vi "数值至码管数组转换.vi"(9 "小数位数":u8, 10 "显示位数":u8=6, 11 "数值":dbl format="%06.3f") -> (3 "数组":u16[](array[numeric]))   [LabVIEW 2013, in "数码管.xctl"]
panel:
  out "子字符串":string
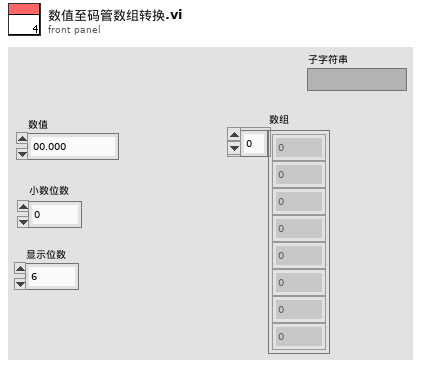
[diagram p1: front panel]
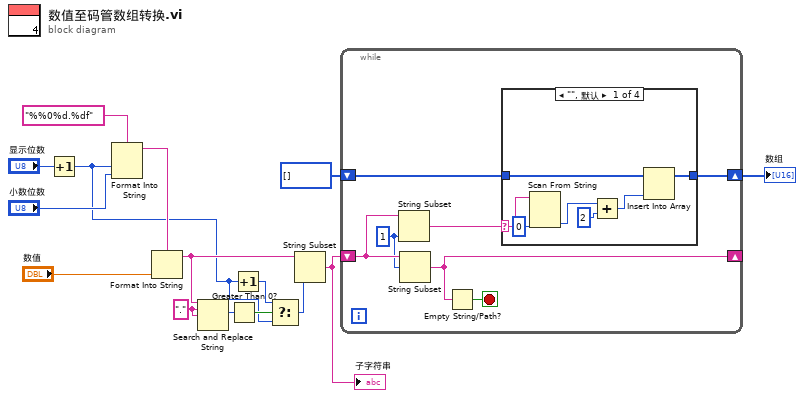
[diagram p0: block diagram]
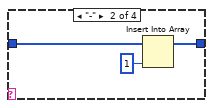
[diagram p2: hidden frame]
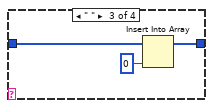
[diagram p3: hidden frame]
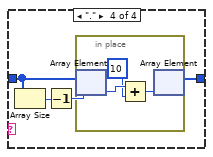
[diagram p4: hidden frame]
diagram:
  w7 = "." ("搜索字符串")
  n1 = Increment(x="显示位数") -> (x+1=w1:u8)
  n2 = Format Into String(format string="%%0%d.%df" ("格式字符串"), w1, "小数位数") -> (resulting string=w12:string)  [unwired: 2 in, 1 out]
  n3 = Format Into String(format string=w12, "数值") -> (resulting string=w8:string)  [unwired: 2 in, 1 out]
  n4 = Search and Replace String(input string=w8, search string=w7, replace string=w7) -> (number of replacements=w6:i32)  [unwired: 5 in, 3 out]
  n5 = Greater Than 0?(x=w6) -> (x > 0?=w5:bool)
  n6 = Increment(x=w1) -> (x+1=w4:u8)
  n7 = Select(t=w4, s=w5, f=w1) -> (s? t:f=w2:u8)
  n8 = String Subset(string=w8, length (rest)=w2) -> (substring=w10:string)  [unwired: 1 in]
  "子字符串" <- w10
  n9 = while {
    shift-right: [w20] -> _
    shift-left: w10 -> [w22]
    shift-right: [w16] -> w9
    shift-left: u16[] [] ("数组") -> [w17]
    stop <- w18 stop-if-true
    w21 = 1 ("长度（剩余）")
    n10 = String Subset(string=w22, length (rest)=w21) -> (substring=w19:string)  [unwired: 1 in]
    n11 = String Subset(string=w22, offset (0)=w21) -> (substring=w20:string)  [unwired: 1 in]
    n12 = Empty String/Path?(string/path=w20) -> (empty?=w18:bool)
    n13 = case shown="\"\", 默认" w19 {
      selector: w19 -> [w29 _ _ _]
      tunnel: w17 -> [w27 w32 w35 w39]
      tunnel: [w26 w31 w34 w36] -> w16
      frame "", Default {
        n14 = Scan From String(input string=w29, default 1=u16 0) -> (output 1=w25:u16)  [unwired: 3 in, 3 out]
        n15 = Add(x=w25, y=u16 2) -> (x+y=w23:u16)
        n16 = Insert Into Array(array=w27, new element=w23) -> (w26:u16[])  [unwired: 1 in]
      }
      frame "-" {
        n17 = Insert Into Array(array=w32, new element=u16 1 ("新元素/子数组")) -> (w31:u16[])  [unwired: 1 in]
      }
      frame " " {
        n18 = Insert Into Array(array=w35, new element=u16 0 ("新元素/子数组")) -> (w34:u16[])  [unwired: 1 in]
      }
      frame "." {
        n19 = Array Size(array=w39) -> (size(s)=w38:i32)
        n20 = Decrement(x=w38) -> (x-1=w37:i32)
        n21 = in-place {
          n22 = in-place-array #1(w39, w37) -> (w42:u16)
          n23 = Add(x=w42, y=u16 10) -> (x+y=w41:u16)
          n24 = in-place-array #1(w41) -> (w36:u16[])  [unwired: 1 out]
        }
      }
    }
  }
  "数组" <- w9
